vi "PV_Gnl_DynamicallyStopEventWhileLoop.vi"(8 "error in":errorcluster, 11 "ViRefNum":refnum<vi>) -> (0 "error out":errorcluster, 3 "ViRefNumDuplicated":refnum<vi>)   [LabVIEW 2020]
doc: "Fonction :\n\nArrête dynamiquement une boucle while.\nGénère un événement utilisateur dynamique de type booléen, relié à la commande Stop du VI référencé.\nTypiquement, ce VI peut arrêter à distance, et proprement, le VI référencé.\nNB : Ce Vi s'exécute même si une erreur est passée en entrée\n\n\n\n*****\n\nEntrées :\n\nVIRefNum : référence du VI. Dupliquée en cas d'erreur. Cette connexion est nécessaire.\n\nerror in : entrée d'erreur.\n\n*****\n\nSorties :\n\nVIRefNumDuplicated : référence du VI.\n\nerror out : sortie d'erreur."
panel:
  # "Input"
  # "Output"
  # "Local"
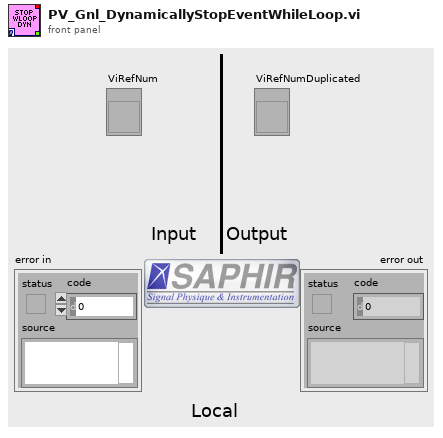
[diagram p1: front panel]
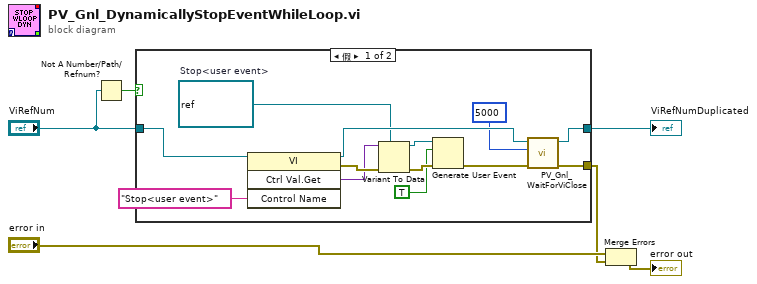
[diagram p0: block diagram]
diagram:
  n1 = Not A Number/Path/Refnum?(number/path/refnum="ViRefNum") -> (NaN/Path/Refnum?=w4:bool)
  n2 = case shown="假" w4 {
    tunnel: "ViRefNum" -> [w16 w20]
    tunnel: [w9 _] -> w2
    tunnel: [w11 w20] -> w5
    frame False {
      w7 = refnum<user-event> refnum  # Stop<user event>
      n3 = invoke class="VI" method="Ctrl Val.Get"(reference=w16, "Control Name"="Stop<user event>") -> (reference out=w12:refnum<vi>, error out=w19:errorcluster, "Get Control Value Variant"=w18:variant)  [unwired: 2 in, 1 out]
      n4 = Variant To Data(error in=w19, type=w7, Variant=w18) -> (data=w14:refnum<user-event>, error out=w15:errorcluster)
      n5 = Generate User Event(user event=w14, event data cluster=TRUE, error in=w15) -> (error out=w10:errorcluster)  [unwired: 1 in, 1 out]
      n6 = call "PV_Gnl_WaitForViClose.vi"("error in"=w10, "TimeOut (ms)"=5000, "ViRefNum"=w12) -> ("error out"=w9:errorcluster, "ViRefNumDuplicated"=w11:refnum<vi>)  [unwired: 7 out]
    }
    frame True {
    }
  }
  "ViRefNumDuplicated" <- w5
  n7 = Merge Errors("error in", w2) -> (→"error out":errorcluster)
